vi "MaskImage.vi"   [LabVIEW 2010]
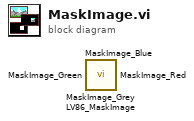
[diagram p0: block diagram]
diagram:
  n1 = call <userlib>:"MaskImage_Grey.vi"() -> ()  [unwired: 3 in, 1 out]
  n2 = call <userlib>:"MaskImage_Blue.vi"() -> ()  [unwired: 3 in, 1 out]
  n3 = call <userlib>:"MaskImage_Green.vi"() -> ()  [unwired: 3 in, 1 out]
  n4 = call <userlib>:"MaskImage_Red.vi"() -> ()  [unwired: 3 in, 1 out]
  n5 = call <userlib>:"LV86_MaskImage.vi"() -> ()  [unwired: 3 in, 1 out]
